vi "Client TX Routing.vi"(8 "error in (no error)":errorcluster, 11 "TCPMessaging in":refnum<class "TCPMessaging.lvclass">) -> (0 "error out":errorcluster)   [LabVIEW 2020, in "Vecto.lvlib" / "TCPMessaging.lvclass"]
doc: "Routes outgoing payloads to the correct client."
uses:
  TCPMessaging.lvclass
  TCPMessaging.lvclass/TCPMessaging.ctl
  SequenceCountService/SequenceCountService.lvclass
  Vecto.lvlib
  proto/TcpPayload/TcpPayload.lvlib
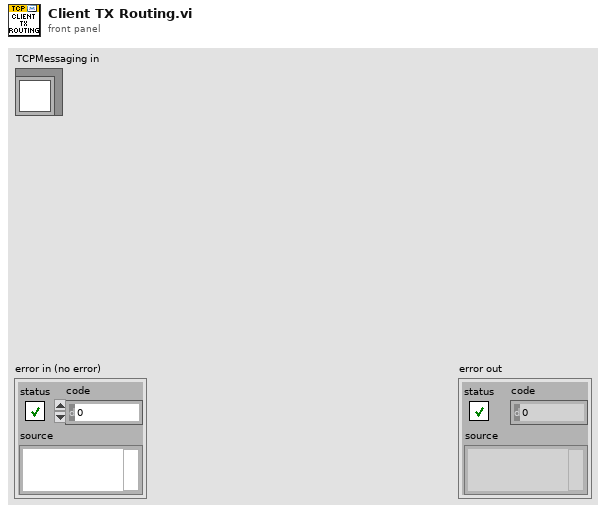
[diagram p1: front panel]
types:
  T1 = typedef "Vecto.lvlib/TX Payload.ctl" = cluster{"Target ID":u32, "Payload":string}
  T2 = typedef "TcpPayload.lvlib/Data.ctl" = cluster{"target_node":u32, "target_task":u32, "source_id":u32, "sequence":u32, "timestamp":u64, "type_id":u32, "payload":u8[]}
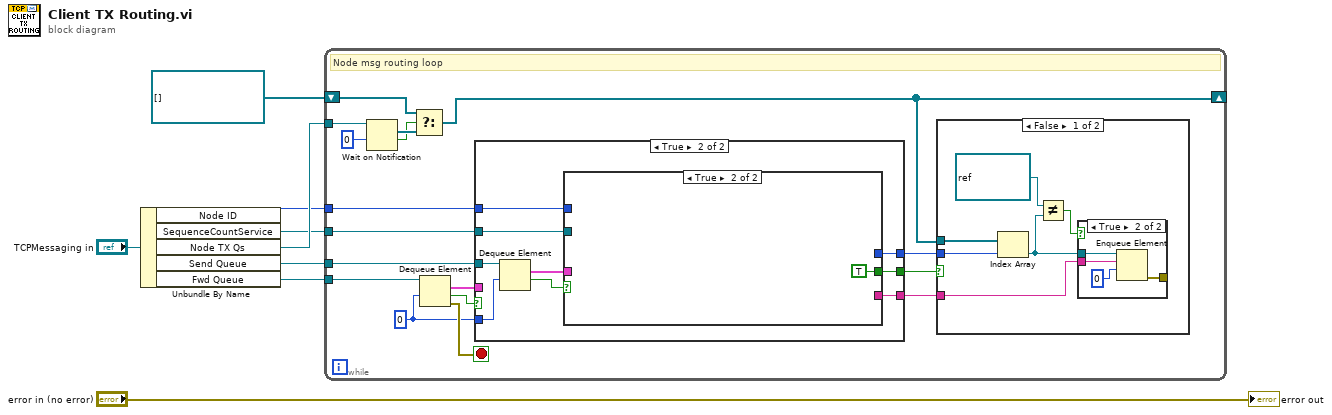
[diagram p0: block diagram]
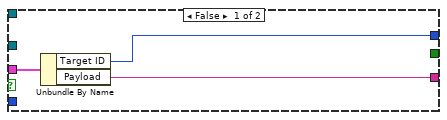
[diagram p4: hidden frame]
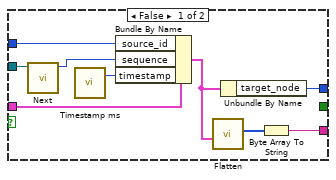
[diagram p5: hidden frame]
diagram:
  n1 = Unbundle By Name("TCPMessaging in") -> ("Node ID"=w2:u32, "SequenceCountService"=w1:refnum<class "SequenceCountService.lvclass">, "Node TX Qs"=w5:refnum<notifier>, "Send Queue"=w6:refnum<queue>, "Fwd Queue"=w3:refnum<queue>)
  n2 = while {
    tunnel: w6 -> [w24]
    tunnel: w5 -> [w23]
    shift-right: [w10] -> _
    shift-left: refnum<queue>[] [] ("queue out") -> [w19]
    tunnel: w3 -> [w18]
    tunnel: w2 -> [w13]
    tunnel: w1 -> [w12]
    stop <- w25 stop-if-true
    w17 = 0 ("timeout in ms (-1)")
    # "Node msg routing loop"
    n3 = Wait on Notification(notifier=w23, timeout in ms (-1)=0) -> (notification=w21:refnum<queue>[], timed out?=w20:bool)  [unwired: 2 in, 2 out]
    n4 = Select(t=w19, s=w20, f=w21) -> (s? t:f=w10:refnum<queue>[])
    n5 = Dequeue Element(queue=w18, timeout in ms (-1)=w17) -> (element=w15:T1, timed out?=w16:bool, error out=w25:errorcluster)  [unwired: 1 in, 1 out]
    n6 = case shown="True" w16 {
      tunnel: w24 -> [_ w47]
      tunnel: w17 -> [_ w45]
      tunnel: w15 -> [w38 _]
      tunnel: [w37 w40] -> w14
      tunnel: w13 -> [_ w43]
      tunnel: w12 -> [_ w42]
      tunnel: [w36 w41] -> w11
      tunnel: [_ w39] -> w9
      frame False {
        n7 = Unbundle By Name(w38) -> ("Target ID"=w37:u32, "Payload"=w36:string)
      }
      frame True {
        n8 = Dequeue Element(queue=w47, timeout in ms (-1)=w45) -> (element=w46:T2, timed out?=w44:bool)  [unwired: 1 in, 2 out]
        n9 = case shown="True" w44 {
          tunnel: w46 -> [w56 _]
          tunnel: w43 -> [w55 _]
          tunnel: w42 -> [w54 _]
          tunnel: [w51 _] -> w41
          tunnel: [w48 _] -> w40
          tunnel: [_ TRUE] -> w39
          frame False {
            n10 = call "Next.vi"("SequenceCountService in"=w54) -> ("Sequence"=w53:u32)  [unwired: 9 in, 1 out]
            n11 = call "Timestamp ms.vi"() -> ("Timestamp ms"=w52:u64)  [unwired: 7 in]
            n12 = Bundle By Name(cluster=w56, "source_id"=w55, "sequence"=w53, "timestamp"=w52) -> (w49:T2)
            n13 = call "Flatten.vi"("Data"=w49) -> ("Buffer"=w50:u8[])  [unwired: 9 in, 1 out]
            n14 = Unbundle By Name(w49) -> ("target_node"=w48:u32)
            n15 = Byte Array To String(unsigned byte array=w50) -> (string=w51:string)
          }
          frame True {
          }
        }
      }
    }
    n16 = case shown="False" w9 {
      tunnel: w14 -> [w29 _]
      tunnel: w11 -> [w28 _]
      tunnel: w10 -> [w26 _]
      frame False {
        n17 = Index Array(array=w26, index=w29) -> (element=w31:refnum<queue>)
        n18 = Not Equal?(x=refnum<queue> refnum ("queue out"), y=w31) -> (x != y?=w27:bool)
        n19 = case shown="True" w27 {
          tunnel: w28 -> [_ w35]
          tunnel: w31 -> [_ w34]
          tunnel: [_ w32] -> _
          frame False {
          }
          frame True {
            n20 = Enqueue Element(queue=w34, element=w35, timeout in ms (-1)=0) -> (error out=w32:errorcluster)  [unwired: 1 in, 2 out]
          }
        }
      }
      frame True {
        # "Sending message is skipped"
      }
    }
  }
  "error out" <- "error in (no error)"
